vi "Three 8-bit Ports Digital Output.vi"(2 "Packet":u64, 4 "Three 8-bit DO Ports":T1={"8-bit DO Port0"="Chassis1/Mod3/DO7:0", "8-bit DO Port1"="Chassis1/Mod3/DO7:0", "8-bit DO Port2"="Chassis1/Mod3/DO7:0"}) -> ()   [LabVIEW 2009]
uses:
  <vilib>/eio/EIONode/EIONode.xnode
  <vilib>/rvi/eio/nirviEIOImplementation/nirviEIOImplementation.xnode
  <vilib>/rvi/eio/common/nirviEmuTemplateMethod_noerrors.vi
  <vilib>/rvi/eio/common/nirviEmuClasses.ctl
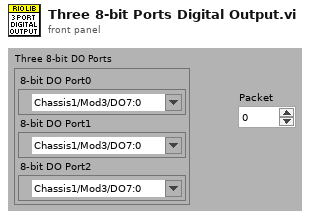
[diagram p1: front panel]
types:
  T1 = cluster{"8-bit DO Port0":refnum<k21>, "8-bit DO Port1":refnum<k21>, "8-bit DO Port2":refnum<k21>}
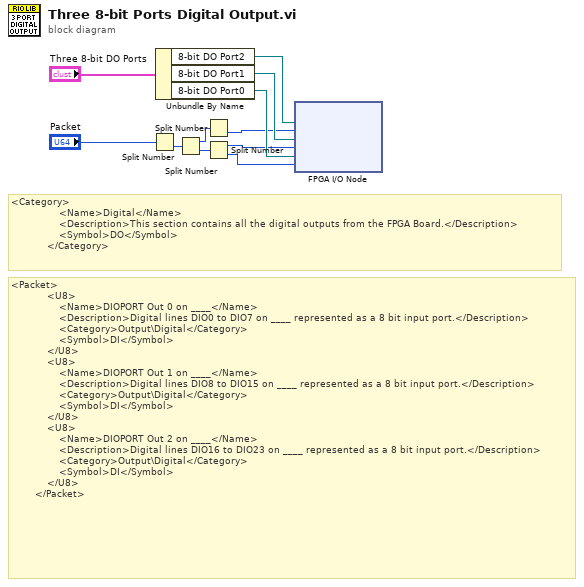
[diagram p0: block diagram]
diagram:
  # "<Packet>\n            <U8>\n                <Name>DIOPORT Out 0 on ____</Name>\n                <Description>Digital lines DIO0 to DIO7 on ____ represented as a 8 bit input port.</Description>\n                <Category>Output\\Digital</Category>\n                <Symbol>DI</Symbol>\n            </U8>\n            <U8>\n                <Name>DIOPORT Out 1 on ____</Name>\n                <Description>Digital lines DIO8 to DIO15 on ____ represented as a 8 bit input port.</Description>\n                <Category>Output\\Digital</Category>\n                <Symbol>DI</Symbol>\n            </U8>\n            <U8>\n                <Name>DIOPORT Out 2 on ____</Name>\n                <Description>Digital lines DIO16 to DIO23 on ____ represented as a 8 bit input port.</Description>\n                <Category>Output\\Digital</Category>\n                <Symbol>DI</Symbol>\n            </U8>\n        </Packet>"
  # "<Category>\n                <Name>Digital</Name>\n                <Description>This section contains all the digital outputs from the FPGA Board.</Description>\n                <Symbol>DO</Symbol>\n            </Category>"
  n1 = Split Number(x="Packet") -> (lo(x)=w10:u32)  [unwired: 1 out]
  n2 = Unbundle By Name("Three 8-bit DO Ports") -> ("8-bit DO Port2"=w3:refnum<k21>, "8-bit DO Port1"=w6:refnum<k21>, "8-bit DO Port0"=w5:refnum<k21>)
  n3 = Split Number(x=w10) -> (hi(x)=w2:u16, lo(x)=w11:u16)
  n4 = Split Number(x=w2) -> (lo(x)=w1:u8)  [unwired: 1 out]
  n5 = Split Number(x=w11) -> (hi(x)=w4:u8, lo(x)=w9:u8)
  n6 = xnode "FPGA I/O Node"("I/O Item"=w1, "I/O Item"=w4, "I/O Item"=w9, "FPGA I/O In"=w3, "FPGA I/O In"=w6, "FPGA I/O In"=w5) -> ()  [unwired: 3 out]
